vi "API - Stream - Download Digital Input Data.vi"(8 "error in":errorcluster, 11 "DAQiFi Device Properties In":T1) -> (0 "error out":errorcluster, 2 "Digital Inputs":bool[](array[boolean]), 3 "DAQiFi Device Properties Out":T1)   [LabVIEW 2021]
doc: "Download Digital Input Data. The array index is arranged according to DIO channel number."
uses:
  TypeDefs/TypeDef - Cluster of DAQiFi Device Properties.ctl
  TypeDefs/Enum - Connection Type.ctl
  TCP - Asynchronous Read of One JSON Message.vi
  USB - Asynchronous Read of One JSON Message.vi
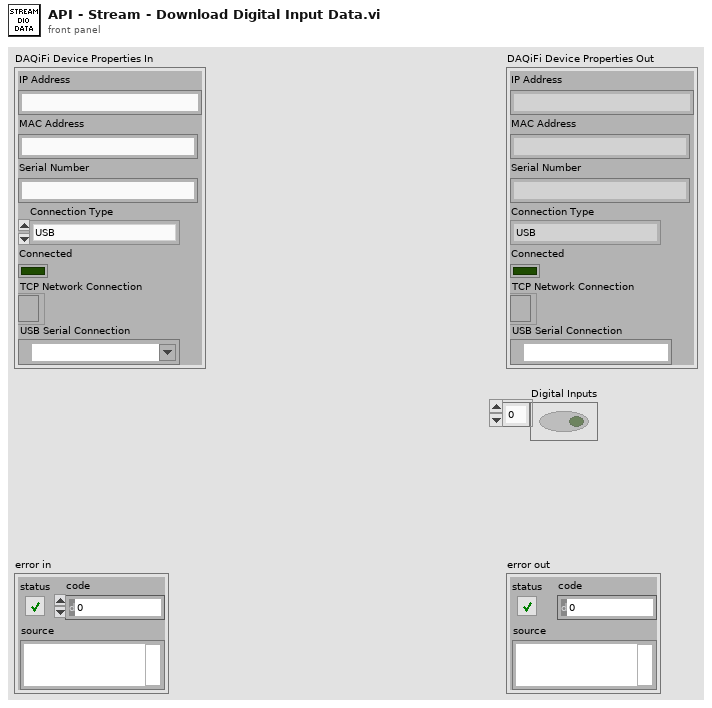
[diagram p1: front panel]
types:
  T1 = typedef "TypeDef - Cluster of DAQiFi Device Properties.ctl" = cluster{"IP Address":string, "MAC Address":string, "Serial Number":string, "Connection Type":T2, "Connected":bool, "TCP Network Connection":refnum<k5>, "USB Serial Connection":refnum<visa-resource-name>}
  T2 = typedef "Enum - Connection Type.ctl" = enum16{"USB", "TCP"}
  T3 = typedef "TypeDef - Cluster Representing Decoded JSON Message.ctl" = cluster{"timestamp":u64, "adc":cluster{"time":i32, "ch":i32, "data":i32}[], "dio":cluster{"time":i32, "mask":i32, "data":u16}[]}
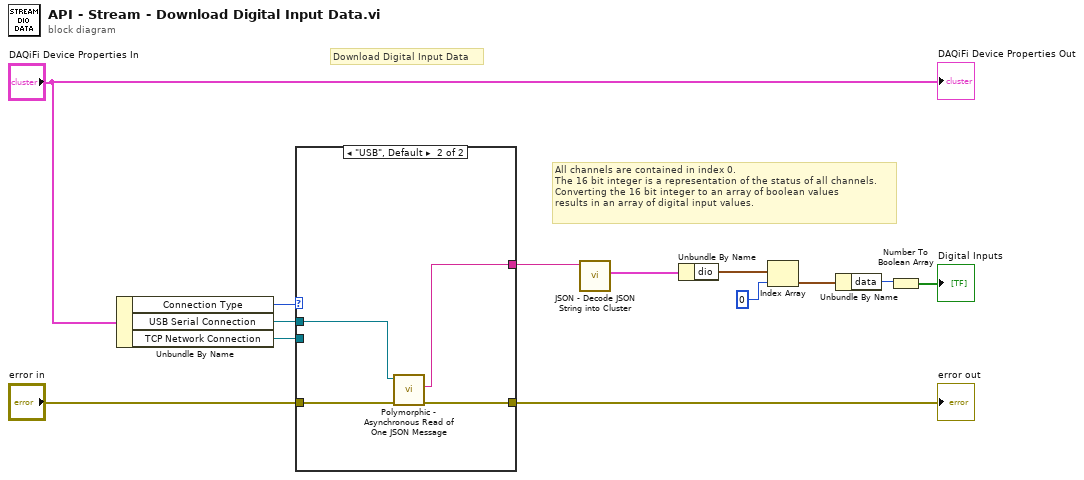
[diagram p0: block diagram]
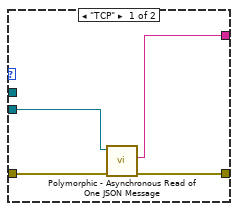
[diagram p2: hidden frame]
diagram:
  # "All channels are contained in index 0.\nThe 16 bit integer is a representation of the status of all channels.\nConverting the 16 bit integer to an array of boolean values \nresults in an array of digital input values."
  # "Download Digital Input Data"
  n1 = Unbundle By Name("DAQiFi Device Properties In") -> ("Connection Type"=w3:T2, "USB Serial Connection"=w1:refnum<visa-resource-name>, "TCP Network Connection"=w2:refnum<k5>)
  n2 = case shown="\"USB\", Default" w3 {
    tunnel: "error in" -> [w17 w21]
    tunnel: [w16 w20] -> w6
    tunnel: [w15 w19] -> w5
    tunnel: w2 -> [w14 _]
    tunnel: w1 -> [_ w18]
    frame "TCP" {
      n3 = call-poly "Polymorphic - Asynchronous Read of One JSON Message.vi"("error in"=w17, "TCP Network Connection in"=w14) -> ("error out"=w16:errorcluster, "Received JSON Message"=w15:string)  [unwired: 7 in, 1 out]
    }
    frame "USB", Default {
      n4 = call-poly "Polymorphic - Asynchronous Read of One JSON Message.vi"("error in"=w21, "VISA resource name in"=w18) -> ("error out"=w20:errorcluster, "Received JSON Message"=w19:string)  [unwired: 7 in, 1 out]
    }
  }
  "error out" <- w6
  n5 = call "JSON - Decode JSON String into Cluster.vi"("JSON String"=w5) -> ("Data out"=w13:T3)  [unwired: 9 in, 1 out]
  n6 = Unbundle By Name(w13) -> ("dio"=w12:cluster{"time":i32, "mask":i32, "data":u16}[])
  n7 = Index Array(array=w12, index=0) -> (element=w10:cluster{"time":i32, "mask":i32, "data":u16})
  n8 = Unbundle By Name(w10) -> ("data"=w9:u16)
  n9 = Number To Boolean Array(number=w9) -> (Boolean array=→"Digital Inputs":bool[])
  "DAQiFi Device Properties Out" <- "DAQiFi Device Properties In"
